vi "writeROTBias.vi"(8 "error in (no error)":errorcluster, 10 "ILC in":refnum<class "ILC.lvclass">, 11 "SingleCylinderActuator in":refnum<class "SingleCylinderActuator.lvclass">) -> (0 "error out":errorcluster, 2 "ILC out":refnum<class "ILC.lvclass">, 3 "SingleCylinderActuator out":refnum<class "SingleCylinderActuator.lvclass">)   [LabVIEW 2015, in "SingleCylinderActuator.lvclass"]
uses:
  SingleCylinderActuator.lvclass
  <userlib>/Common/ILC/ILC/ILC.lvclass
  SingleCylinderActuator.lvclass/SingleCylinderActuator.ctl
  <userlib>/Common/ILC/ILC/ILC.lvclass/ILC.ctl
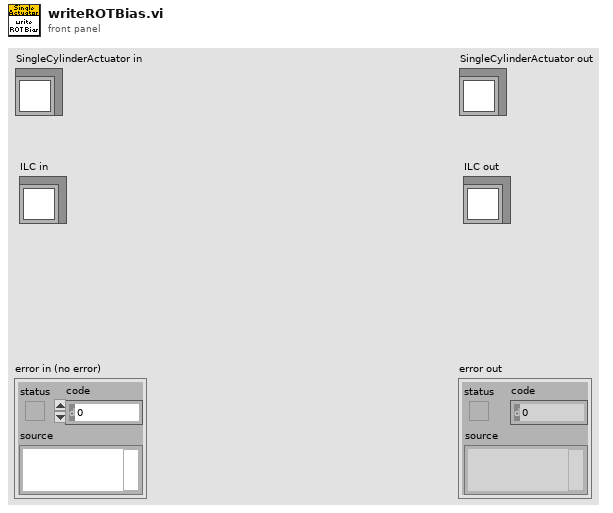
[diagram p1: front panel]
types:
  T1 = typedef "ILCCommon.lvlib/ILCTypedefs.lvlib/Outputs.ctl" = cluster{"Step & Direction":i16, "Blower RPM":u8, "PWM (SSR)":u8, "Ch1":u16, "Ch2":u16, "Ch3":u16, "Ch4":u16}
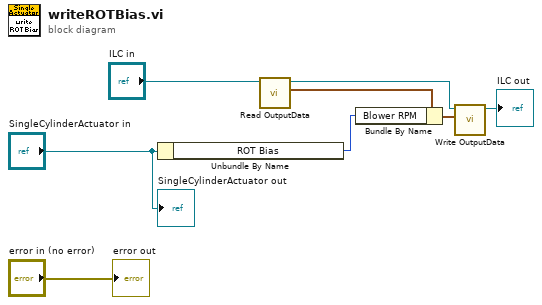
[diagram p0: block diagram]
diagram:
  n1 = Unbundle By Name("SingleCylinderActuator in") -> ("ROT Bias"=w3:u8)
  n2 = call <userlib>:"Read OutputData.vi"("ILC in"="ILC in") -> ("OutputData"=w6:T1, "ILC out"=w4:refnum<class "ILC.lvclass">)  [unwired: 9 in]
  n3 = Bundle By Name(cluster=w6, "Blower RPM"=w3) -> (w5:T1)
  n4 = call <userlib>:"Write OutputData.vi"("OutputData"=w5, "ILC in"=w4) -> ("ILC out"=→"ILC out":refnum<class "ILC.lvclass">)  [unwired: 9 in]
  "error out" <- "error in (no error)"
  "SingleCylinderActuator out" <- "SingleCylinderActuator in"
